vi "DPID Dialog.vi"(8 "error in (no error)":errorcluster, 9 "Existing DPIDs":u8[](array[numeric]), 10 "Existing PIDs":T1[](array[typedef]) {"Signals"."Byte Order" items=["Little Endian", "Big Endian"]; "Signals"."Data Type" items=["Signed", "Unsigned", "IEEE Float"]}, 11 "DPID":T4) -> (0 "error out":errorcluster, 2 "Cancel PID?":bool, 3 "DPID":T4)   [LabVIEW 2015, in "Diagnostics Addon System Explorer.lvlib"]
uses:
  Diagnostics Addon System Explorer.lvlib
  Shared/Types/DPID Periodic Rate.ctl
  Shared/Types/DPID Parameters.ctl
  Shared/Types/Frame Parameters.ctl
  Shared/Types/Signal Parameters.ctl
  <vilib>/NI/AMC/Read Termination Message.vi
  <vilib>/NI/AMC/Create Single Message.vi
  <vilib>/NI/AMC/Update Message Routing Info.vi
  <vilib>/NI/AMC/Globals.vi
  <vilib>/NI/AMC/Send Message.vi
  <vilib>/NI/AMC/AMC.lvlib
  Shared/Diagnostics Addon Shared.lvlib
panel:
  in  "Remove":bool
  in  "Speed":T3
  in  "DPID ID":u8=1 min=1 format="%.0x"
  in  "Add":bool
  in  "PID":string(combo)
  in  "PIDs":i32(listbox)
  in  "Cancel PID":bool
  in  "Apply":bool
  in  "Cancel":bool
  in  "OK":bool
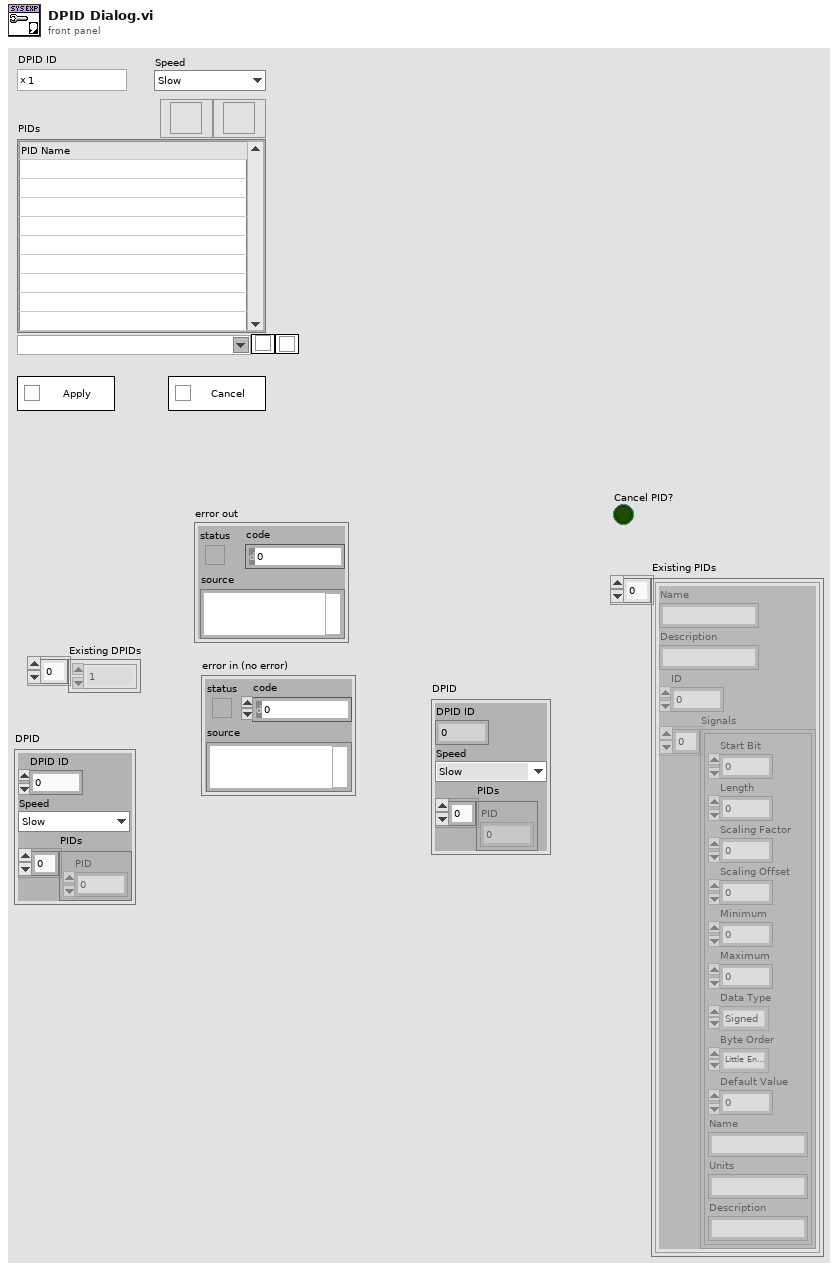
[diagram p1: front panel]
types:
  T1 = typedef "Diagnostics Addon Shared.lvlib/Frame Parameters.ctl" = cluster{"Name":string, "Description":string, "ID":u32, "Signals":T2[]}
  T2 = typedef "Diagnostics Addon Shared.lvlib/Signal Parameters.ctl" = cluster{"Start Bit":u8, "Length":u8, "Scaling Factor":dbl, "Scaling Offset":dbl, "Minimum":dbl, "Maximum":dbl, "Data Type":u32, "Byte Order":u32, "Default Value":dbl, "Name":string, "Units":string, "Description":string}
  T3 = typedef "Diagnostics Addon Shared.lvlib/DPID Periodic Rate.ctl" = enum16{"Slow", "Medium", "Fast"}
  T4 = typedef "Diagnostics Addon Shared.lvlib/DPID Parameters.ctl" = cluster{"DPID ID":u8, "Speed":T3, "PIDs":u16[]}
  T5 = cluster{"NewControlRefs":refnum<vi>[], "Add":refnum<vi>, "Listbox":refnum<vi>, "Remove":refnum<vi>, "Apply":refnum<vi>, "Cancel PID":refnum<vi>}
  T6 = typedef "AMC.lvlib/Message Queue.ctl" = refnum<queue>
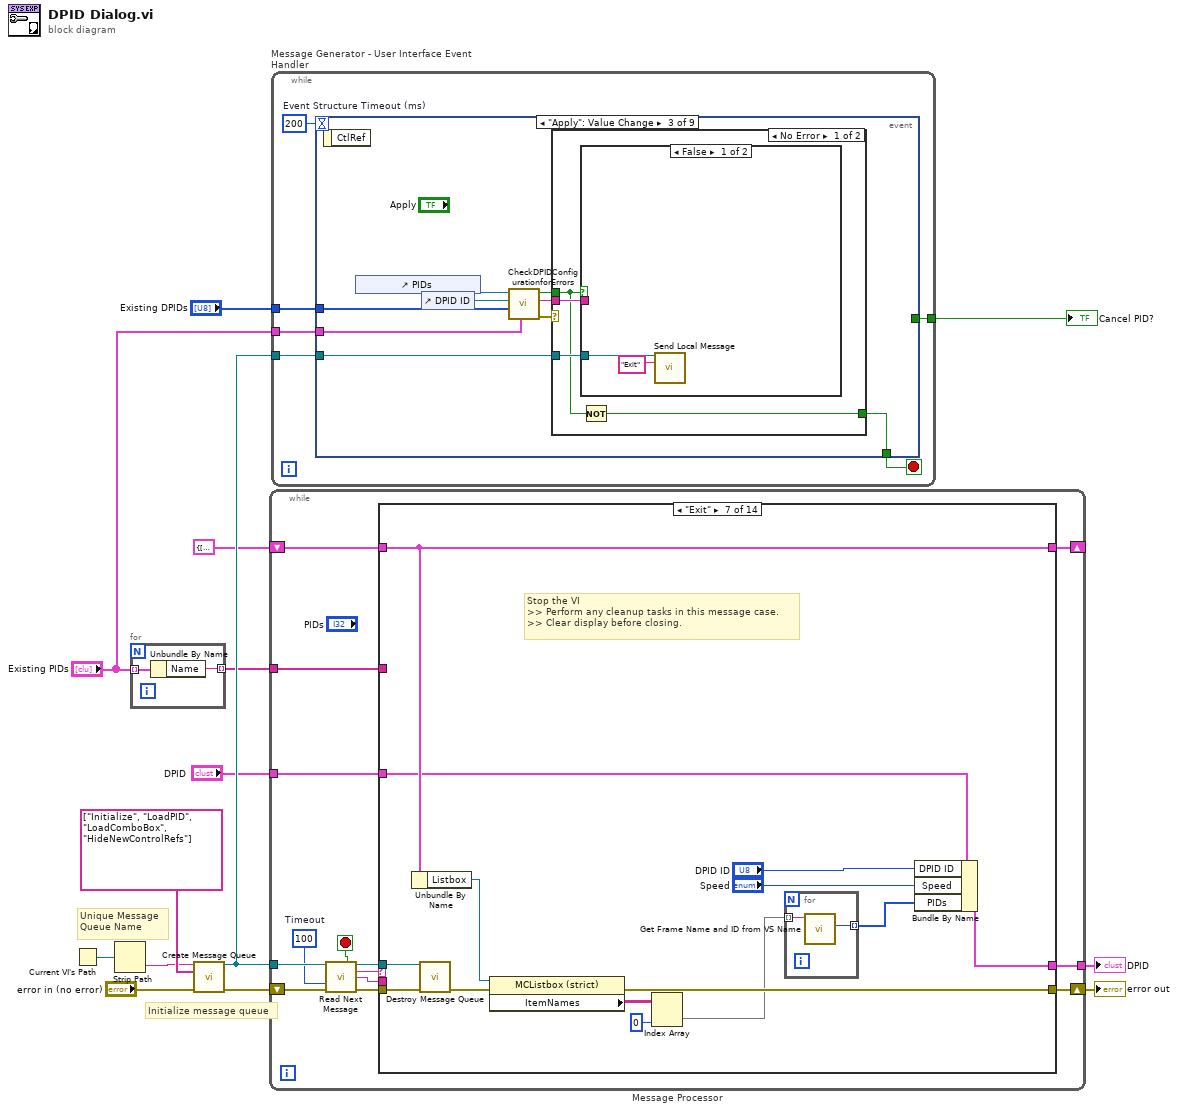
[diagram p0: block diagram]
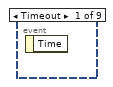
[diagram p2: hidden frame]
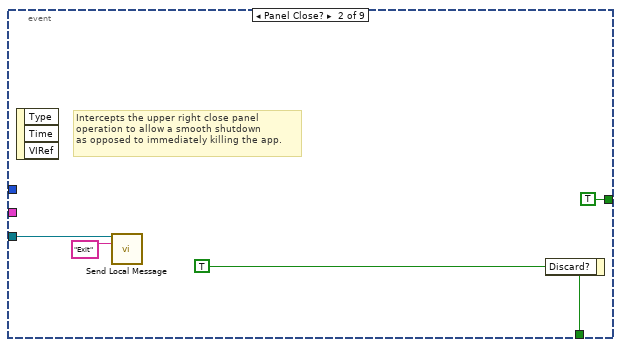
[diagram p3: hidden frame]
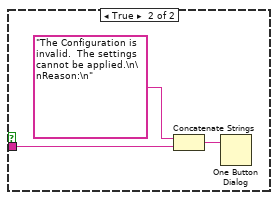
[diagram p4: hidden frame]
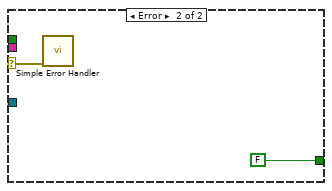
[diagram p5: hidden frame]
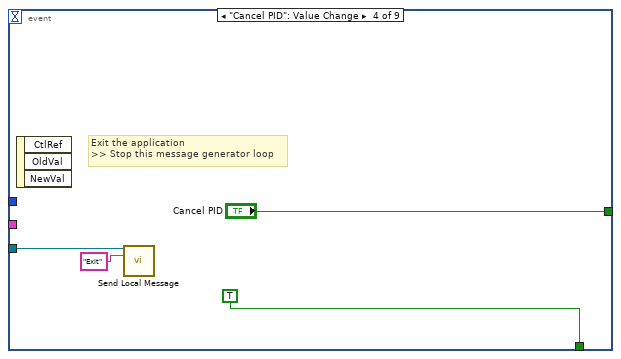
[diagram p6: hidden frame]
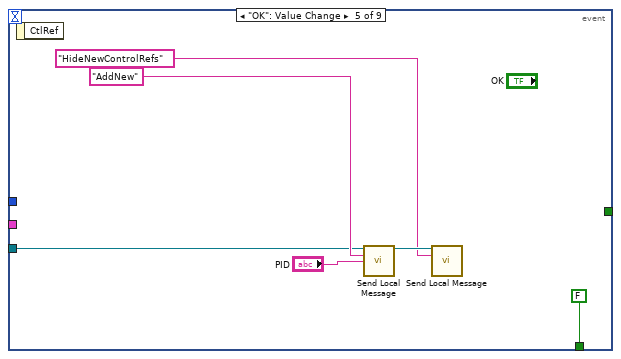
[diagram p7: hidden frame]
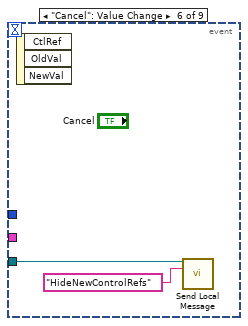
[diagram p8: hidden frame]
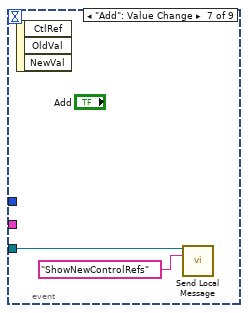
[diagram p9: hidden frame]
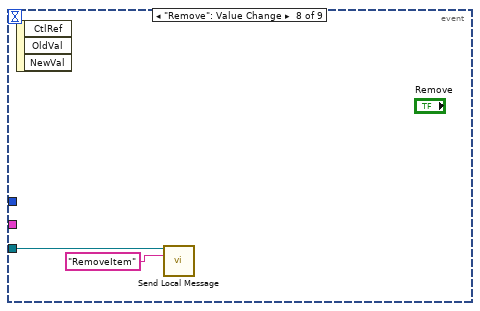
[diagram p10: hidden frame]
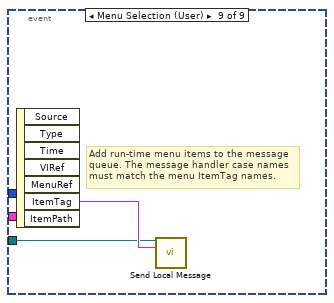
[diagram p11: hidden frame]
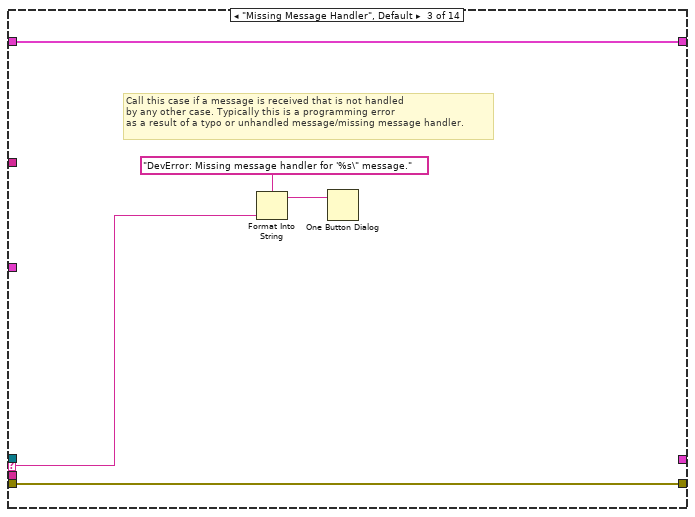
[diagram p14: hidden frame]
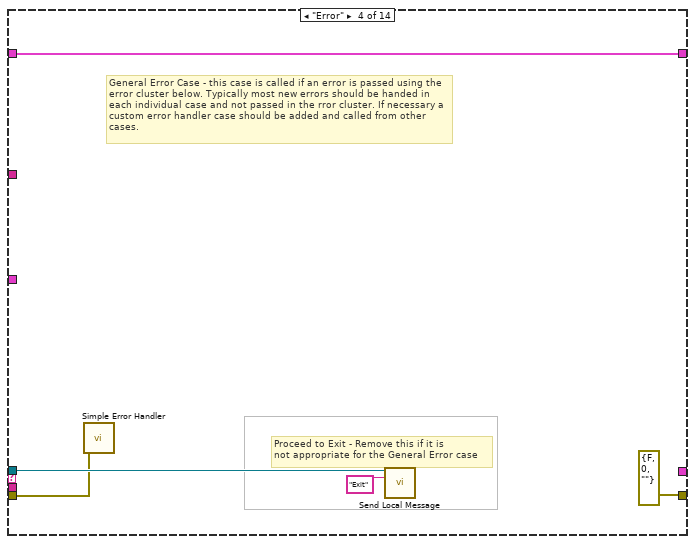
[diagram p15: hidden frame]
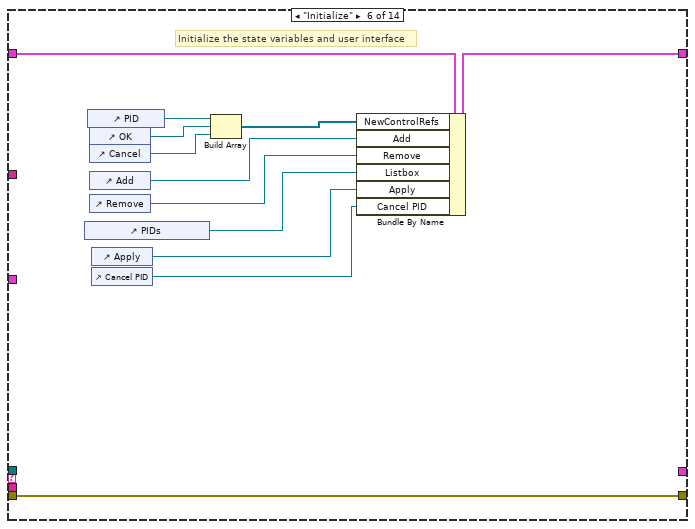
[diagram p17: hidden frame]
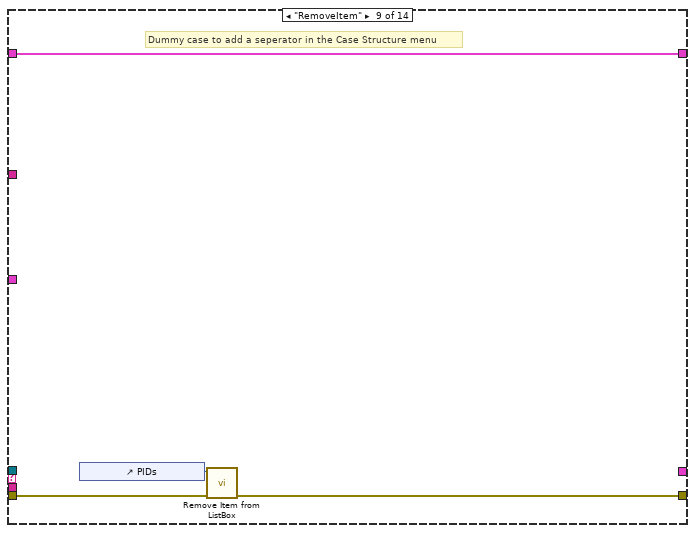
[diagram p19: hidden frame]
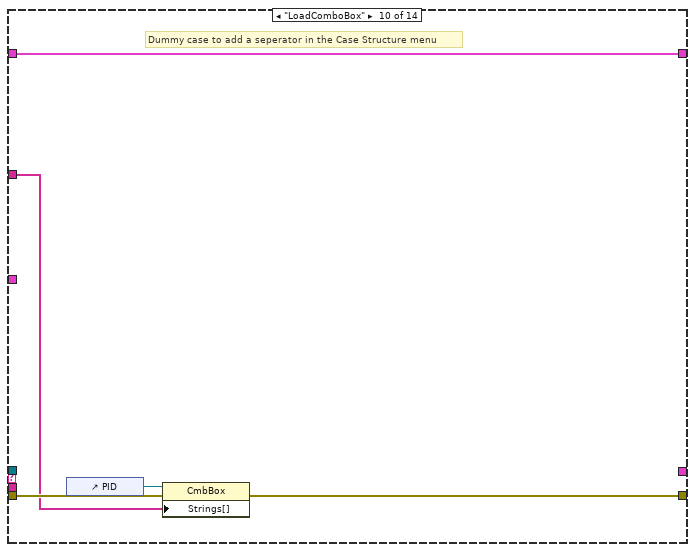
[diagram p20: hidden frame]
diagram:
  # "Initialize message queue"
  # "Unique Message\nQueue Name"
  n1 = Current VI's Path() -> (path=w10:path)
  n2 = Strip Path(path=w10) -> (name=w13:string)  [unwired: 1 out]
  n3 = for {
    tunnel: "Existing PIDs" -> [w16] mode=indexing
    tunnel: [w15] -> w2 mode=indexing
    n4 = Unbundle By Name(w16) -> ("Name"=w15:string)
  }
  n5 = call <vilib>:"Create Message Queue.vi"("message queue name"=w13, "initial message names"=string[] ["Initialize", "LoadPID", "LoadComboBox", "HideNewControlRefs"], "error in"="error in (no error)") -> ("message queue out"=w12:T6, "error out"=w11:errorcluster)  [unwired: 11 in]
  n6 = while "Message Processor" {
    shift-left: w11 -> [w24]
    shift-right: [w28] -> w5
    tunnel: w12 -> [w25]
    shift-left: T5 {"NewControlRefs"=[], "Add"=refnum, "Listbox"=refnum, "Remove"=refnum, "Apply"=refnum, "Cancel PID"=refnum} ("State Variables") -> [w30]
    shift-right: [w29] -> _
    tunnel: [w19] -> w7
    tunnel: "DPID" -> [w18]
    tunnel: w2 -> [w17]
    stop <- w27 stop-if-true
    w22 = 100  # Timeout
    n7 = call <vilib>:"Read Next Message.vi"("message queue in"=w25, "timeout (1 ms)"=w22, "error in"=w24) -> ("exit process?"=w27:bool, "message queue out"=w26:T6, "message name"=w21:string, "message value"=w20:string, "error out"=w23:errorcluster)  [unwired: 5 in, 3 out]
    n8 = case shown="\"Exit\"" w21 {
      selector: w21 -> [_ _ w37 _ _ _ _ _ _ _ _ _ _ _]
      tunnel: [w32 w34 w39 w44 w46 w53 w70 w76 w80 w85 w103 w123 w137 w152] -> w29
      tunnel: w30 -> [w32 w34 w39 w44 w46 w54 w70 w76 w80 w85 w103 w123 w137 w152]
      tunnel: w26 -> [_ _ _ w42 _ _ w71 _ _ _ _ _ _ _]
      tunnel: w23 -> [w31 w33 w38 w40 w45 w51 w72 w75 w78 w83 w97 w120 w136 w151]
      tunnel: [w31 w33 w38 errorcluster {"status"=FALSE, "code"=0, "source"=""} ("error out") w45 w51 w63 w75 w77 w82 w96 w121 w127 w140] -> w28
      tunnel: w20 -> [_ _ _ _ _ _ _ _ _ _ _ w119 _ _]
      tunnel: [_ _ _ _ _ _ w66 _ _ _ _ _ _ _] -> w19
      tunnel: w18 -> [_ _ _ _ _ _ w65 _ _ _ w95 _ _ _]
      tunnel: w17 -> [_ _ _ _ _ _ _ _ _ w81 w86 _ _ _]
      frame "---------- Framework Operations ----------" {
        # "Dummy case to add a seperator in the Case Structure menu"
      }
      frame "", "Idle" {
        # "Idle Case - this case is called after a Timeout on the Get Next Message from Queue VI, if no new messages are present on the queue. This case can be used for housekeeping tasks such as updating the UI."
      }
      frame "Missing Message Handler", Default {
        # "Call this case if a message is received that is not handled \nby any other case. Typically this is a programming error\nas a result of a typo or unhandled message/missing message handler."
        n9 = Format Into String(format string="DevError: Missing message handler for '%s\" message." ("message"), w37) -> (resulting string=w35:string)  [unwired: 2 in, 1 out]
        n10 = One Button Dialog(message=w35) -> ()  [unwired: 2 out]
      }
      frame "Error" {
        # "Proceed to Exit - Remove this if it is\nnot appropriate for the General Error case"
        # "General Error Case - this case is called if an error is passed using the error cluster below. Typically most new errors should be handed in each individual case and not passed in the rror cluster. If necessary a custom error handler case should be added and called from other cases."
        n11 = call <vilib>:"Simple Error Handler.vi"("error in (no error)"=w40) -> ()  [unwired: 1 in, 8 out]
        n12 = call <vilib>:"Send Local Message.vi"("message queue in"=w42, "message name"="Exit") -> ()  [unwired: 11 in, 3 out]
      }
      frame "---------- Generic Operations ----------" {
        # "Dummy case to add a seperator in the Case Structure menu"
      }
      frame "Initialize" {
        # "Initialize the state variables and user interface"
        n13 = control-ref of="PIDs"() -> (w52:refnum<vi>)
        n14 = control-ref of="PID"() -> (w56:refnum<vi>)
        n15 = control-ref of="OK"() -> (w57:refnum<vi>)
        n16 = control-ref of="Cancel"() -> (w58:refnum<vi>)
        n17 = control-ref of="Add"() -> (w50:refnum<vi>)
        n18 = control-ref of="Remove"() -> (w49:refnum<vi>)
        n19 = control-ref of="Apply"() -> (w48:refnum<vi>)
        n20 = control-ref of="Cancel PID"() -> (w47:refnum<vi>)
        n21 = Build Array(w56, w57, w58) -> (w55:refnum<vi>[])
        n22 = Bundle By Name(cluster=w54, "NewControlRefs"=w55, "Add"=w50, "Remove"=w49, "Listbox"=w52, "Apply"=w48, "Cancel PID"=w47) -> (w53:T5)
      }
      frame "Exit" {
        # "Stop the VI\n>> Perform any cleanup tasks in this message case.\n>> Clear display before closing."
        n23 = Unbundle By Name(w70) -> ("Listbox"=w69:refnum<vi>)
        n24 = call <vilib>:"Destroy Message Queue.vi"("message queue in"=w71, "error in"=w72) -> ("error out"=w68:errorcluster)  [unwired: 11 in, 2 out]
        n25 = property class="MCListbox (strict)"(reference=w69, error in=w68) -> (error out=w63:errorcluster, "ItemNames"=w64:string[][])  [unwired: 1 out]
        n26 = Index Array(array=w64, index (col)=0 ("disabled index (col)")) -> (element=w59:string[])  [unwired: 1 in]
        n27 = for {
          tunnel: w59 -> [w73] mode=indexing
          tunnel: [w74] -> w60 mode=indexing
          n28 = call "Get Frame Name and ID from VS Name.vi"("VS PID Name"=w73) -> ("ID"=w74:u16)  [unwired: 9 in, 1 out]
        }
        n29 = Bundle By Name(cluster=w65, "DPID ID"="DPID ID", "Speed"="Speed", "PIDs"=w60) -> (w66:T4)
      }
      frame "---------- Application Operations ----------" {
        # "Dummy case to add a seperator in the Case Structure menu"
      }
      frame "RemoveItem" {
        # "Dummy case to add a seperator in the Case Structure menu"
        n30 = control-ref of="PIDs"() -> (w79:refnum<vi>)
        n31 = call "Remove Item from ListBox.vi"("error in (no error)"=w78, "MulticolumnListbox in"=w79) -> ("error out"=w77:errorcluster)  [unwired: 9 in]
      }
      frame "LoadComboBox" {
        # "Dummy case to add a seperator in the Case Structure menu"
        n32 = control-ref of="PID"() -> (w84:refnum<vi>)
        n33 = property class="CmbBox"(reference=w84, error in=w83, "Strings[]"=w81) -> (error out=w82:errorcluster)  [unwired: 1 out]
      }
      frame "LoadPID" {
        # "Dummy case to add a seperator in the Case Structure menu"
        n34 = Unbundle By Name(w95) -> ("PIDs"=w89:u16[], "Speed"=w93:T3, "DPID ID"=w94:u8)
        n35 = for {
          tunnel: w86 -> [w116] mode=indexing
          tunnel: [w117] -> w90 mode=indexing
          n36 = call "Get Frame Name and ID from VS Name.vi"("VS PID Name"=w116) -> ("ID"=w117:u16)  [unwired: 9 in, 1 out]
        }
        n37 = control-ref of="DPID ID"() -> (w99:refnum<vi>)
        n38 = control-ref of="Speed"() -> (w92:refnum<vi>)
        n39 = for {
          tunnel: w90 -> [w108]
          tunnel: w86 -> [w107]
          tunnel: w89 -> [w104] mode=indexing
          tunnel: [w106] -> w88 mode=indexing
          n40 = Search 1D Array(1D array=w108, element=w104) -> (index of element=w105:i32)  [unwired: 1 in]
          n41 = case shown="Default" w105 {
            selector: w105 -> [_ w113]
            tunnel: w107 -> [_ w115]
            tunnel: [w109 w114] -> w106
            tunnel: w104 -> [w112 _]
            frame -1 {
              n42 = Number To Hexadecimal String(2:w112) -> (0:w111:string)  [unwired: 1 in]
              n43 = Concatenate Strings(w111, " - Error: No Matching PID" ("PID Name")) -> (w109:string)
            }
            frame Default {
              n44 = Index Array(array=w115, index=w113) -> (element=w114:string)
            }
          }
        }
        n45 = property class="DigNum (strict)"(reference=w99, error in=w97, "Value"=w94) -> (error out=w100:errorcluster)  [unwired: 1 out]
        n46 = property class="Enum (strict)"(reference=w92, error in=w100, "Value"=w93) -> (error out=w98:errorcluster)  [unwired: 1 out]
        n47 = control-ref of="PIDs"() -> (w102:refnum<vi>)
        n48 = Build Array(w88) -> (w87:string[][])
        n49 = Transpose 2D Array(2D array=w87) -> (transposed array=w91:string[][])
        n50 = property class="MCListbox (strict)"(reference=w102, error in=w98, "ItemNames"=w91, "Value"=0) -> (error out=w96:errorcluster)  [unwired: 1 out]
      }
      frame "AddNew" {
        # "Dummy case to add a seperator in the Case Structure menu"
        n51 = Build Array(w119) -> (w118:string[])
        n52 = Unbundle By Name(w123) -> ("Listbox"=w122:refnum<vi>)
        n53 = call "Add Item to Listbox.vi"("error in (no error)"=w120, "Item"=w118, "MulticolumnListbox in"=w122) -> ("error out"=w121:errorcluster)  [unwired: 8 in]
      }
      frame "HideNewControlRefs" {
        w124 = TRUE ("Visible")
        # "Dummy case to add a seperator in the Case Structure menu"
        n54 = Unbundle By Name(w137) -> ("Cancel PID"=w125:refnum<vi>, "Apply"=w126:refnum<vi>, "Remove"=w130:refnum<vi>, "Add"=w132:refnum<vi>, "NewControlRefs"=w135:refnum<vi>[])
        n55 = call "Visible Control References.vi"("error in"=w136, "Visible?"=FALSE, "Control Refs"=w135) -> ("error out"=w133:errorcluster)  [unwired: 8 in]
        n56 = property class="Bool"(reference=w132, error in=w133, "Visible"=w124) -> (error out=w131:errorcluster)  [unwired: 1 out]
        n57 = property class="Bool"(reference=w130, error in=w131, "Visible"=w124) -> (error out=w128:errorcluster)  [unwired: 1 out]
        n58 = property class="Bool"(reference=w126, error in=w128, "Visible"=w124) -> (error out=w129:errorcluster)  [unwired: 1 out]
        n59 = property class="Bool"(reference=w125, error in=w129, "Visible"=w124) -> (error out=w127:errorcluster)  [unwired: 1 out]
      }
      frame "ShowNewControlRefs" {
        w143 = FALSE ("Visible")
        w145 = FALSE ("Visible")
        # "Dummy case to add a seperator in the Case Structure menu"
        n60 = Unbundle By Name(w152) -> ("Apply"=w139:refnum<vi>, "Cancel PID"=w138:refnum<vi>, "Remove"=w144:refnum<vi>, "Add"=w147:refnum<vi>, "NewControlRefs"=w150:refnum<vi>[])
        n61 = call "Visible Control References.vi"("error in"=w151, "Visible?"=TRUE, "Control Refs"=w150) -> ("error out"=w148:errorcluster)  [unwired: 8 in]
        n62 = property class="Bool"(reference=w147, error in=w148, "Visible"=w145) -> (error out=w146:errorcluster)  [unwired: 1 out]
        n63 = property class="Bool"(reference=w144, error in=w146, "Visible"=w145) -> (error out=w141:errorcluster)  [unwired: 1 out]
        n64 = property class="Bool"(reference=w138, error in=w141, "Visible"=w143) -> (error out=w142:errorcluster)  [unwired: 1 out]
        n65 = property class="Bool"(reference=w139, error in=w142, "Visible"=w143) -> (error out=w140:errorcluster)  [unwired: 1 out]
      }
    }
  }
  "DPID" <- w7
  "error out" <- w5
  n66 = while "Message Generator - User Interface Event Handler" {
    tunnel: w12 -> [w156]
    tunnel: [w155] -> w8
    tunnel: "Existing DPIDs" -> [w154]
    tunnel: "Existing PIDs" -> [w153]
    stop <- w157 stop-if-true
    w158 = 200  # Event Structure Timeout (ms)
    n67 = event shown="[2] \"Apply\": Value Change" {
      selector: _ -> [_ _ _ _ _ _ _ _ _]
      dyn-events: _ -> [_ _ _ _ _ _ _ _ _]
      timeout: w158 -> [_ _ _ _ _ _ _ _ _]
      tunnel: [_ w162 w163 TRUE ("Discard?") FALSE ("Discard?") _ _ _ _] -> w157
      tunnel: w156 -> [_ w160 w167 w184 w190 w193 w195 w197 w199]
      tunnel: [_ TRUE ("Cancel PID") _ "Cancel PID" _ _ _ _ _] -> w155
      tunnel: w154 -> [_ _ w169 _ _ _ _ _ _]
      tunnel: w153 -> [_ _ w168 _ _ _ _ _ _]
      event Timeout {
        n68 = event-data() -> ()  [unwired: 2 out]
      }
      event Panel Close? {
        w162 = TRUE ("Discard?")
        # "Intercepts the upper right close panel\noperation to allow a smooth shutdown\nas opposed to immediately killing the app."
        n69 = event-data() -> ()  [unwired: 4 out]
        n70 = call <vilib>:"Send Local Message.vi"("message queue in"=w160, "message name"="Exit") -> ()  [unwired: 11 in, 3 out]
        n71 = event-data("Discard?"=w162) -> ()  [unwired: 1 in, 1 out]
      }
      event "Apply": Value Change {
        n72 = event-data() -> ()  [unwired: 2 out]
        n73 = control-ref of="PIDs"() -> (w171:refnum<vi>)
        n74 = control-ref of="DPID ID"() -> (w170:refnum<vi>)
        n75 = call "CheckDPIDConfigurationforErrors.vi"("Existing PIDs"=w168, "Existing DPIDs"=w169, "DPID ID"=w170, "PIDs"=w171) -> ("error out"=w165:errorcluster, "Reason"=w164:string, "Error?"=w166:bool)  [unwired: 5 in]
        n76 = case shown="No Error" w165 {
          selector: w165 -> [_ w182]
          tunnel: w166 -> [w173 _]
          tunnel: w167 -> [w175 _]
          tunnel: w164 -> [w174 _]
          tunnel: [w172 FALSE] -> w163
          frame No Error {
            n77 = case shown="False" w173 {
              tunnel: w175 -> [w177 _]
              tunnel: w174 -> [_ w180]
              frame False {
                n78 = call <vilib>:"Send Local Message.vi"("message queue in"=w177, "message name"="Exit" ("Message Name")) -> ()  [unwired: 11 in, 3 out]
              }
              frame True {
                n79 = Concatenate Strings("The Configuration is invalid.  The settings cannot be applied.\n\nReason:\n" ("message"), w180) -> (w178:string)
                n80 = One Button Dialog(message=w178) -> ()  [unwired: 1 in, 1 out]
              }
            }
            n81 = Not(x=w173) -> (.not. x?=w172:bool)
          }
          frame Error {
            n82 = call <vilib>:"Simple Error Handler.vi"("error in (no error)"=w182) -> ()  [unwired: 4 in, 5 out]
          }
        }
      }
      event "Cancel PID": Value Change {
        # "Exit the application\n>> Stop this message generator loop"
        n83 = event-data() -> ()  [unwired: 4 out]
        n84 = call <vilib>:"Send Local Message.vi"("message queue in"=w184, "message name"="Exit") -> ()  [unwired: 11 in, 3 out]
      }
      event "OK": Value Change {
        n85 = event-data() -> ()  [unwired: 2 out]
        n86 = call <vilib>:"Send Local Message.vi"("message queue in"=w190, "message name"="AddNew", "message value"="PID") -> ("message queue out"=w189:T6)  [unwired: 10 in, 2 out]
        n87 = call <vilib>:"Send Local Message.vi"("message queue in"=w189, "message name"="HideNewControlRefs" ("Message Name")) -> ()  [unwired: 11 in, 3 out]
      }
      event "Cancel": Value Change {
        n88 = event-data() -> ()  [unwired: 4 out]
        n89 = call <vilib>:"Send Local Message.vi"("message queue in"=w193, "message name"="HideNewControlRefs" ("Message Name")) -> ()  [unwired: 11 in, 3 out]
      }
      event "Add": Value Change {
        n90 = event-data() -> ()  [unwired: 4 out]
        n91 = call <vilib>:"Send Local Message.vi"("message queue in"=w195, "message name"="ShowNewControlRefs" ("Message Name")) -> ()  [unwired: 11 in, 3 out]
      }
      event "Remove": Value Change {
        n92 = event-data() -> ()  [unwired: 4 out]
        n93 = call <vilib>:"Send Local Message.vi"("message queue in"=w197, "message name"="RemoveItem") -> ()  [unwired: 11 in, 3 out]
      }
      event Menu Selection (User) {
        # "Add run-time menu items to the message\nqueue. The message handler case names must match the menu ItemTag names."
        n94 = event-data() -> ("ItemTag"=w200:string)  [unwired: 7 out]
        n95 = call <vilib>:"Send Local Message.vi"("message queue in"=w199, "message name"=w200) -> ()  [unwired: 11 in, 3 out]
      }
    }
  }
  "Cancel PID?" <- w8
